vi "GetProperties.vi"(8 "error in":errorcluster, 11 "PageSelector in":refnum<class "PageSelector.lvclass">) -> (0 "error out":errorcluster, 3 "PageSelector out":refnum<class "PageSelector.lvclass">)   [LabVIEW 2014, in "PageSelector.lvclass"]
uses:
  PageSelector.lvclass
  PageSelector.lvclass/PageSelector.ctl
  Control/Control.lvclass
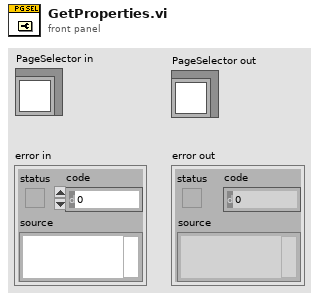
[diagram p1: front panel]
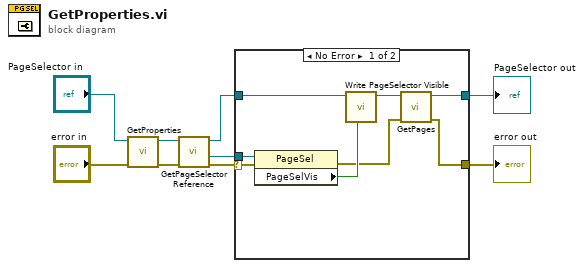
[diagram p0: block diagram]
diagram:
  n1 = call-parent "GetProperties.vi"("error in"="error in", "Control in"="PageSelector in") -> ("error out"=w6:errorcluster, "Control out"=w7:refnum<class "PageSelector.lvclass">)  [unwired: 8 in]
  n2 = call "GetPageSelectorReference.vi"("error in"=w6, "PageSelector in"=w7) -> ("error out"=w5:errorcluster, "page selector reference"=w4:refnum<vi>, "PageSelector out"=w3:refnum<class "PageSelector.lvclass">)  [unwired: 7 in]
  n3 = case shown="No Error" w5 {
    selector: w5 -> [w16 w19]
    tunnel: w4 -> [w15 _]
    tunnel: w3 -> [w17 w18]
    tunnel: [w11 w19] -> w2
    tunnel: [w10 w18] -> w1
    frame No Error {
      n4 = property class="PageSel"(reference=w15, error in=w16) -> (error out=w12:errorcluster, "PageSelVis"=w14:bool)  [unwired: 1 out]
      n5 = call "Write PageSelector Visible.vi"("Visible"=w14, "PageSelector in"=w17) -> ("PageSelector out"=w13:refnum<class "PageSelector.lvclass">)  [unwired: 7 in]
      n6 = call "GetPages.vi"("error in"=w12, "PageSelector in"=w13) -> ("error out"=w11:errorcluster, "PageSelector out"=w10:refnum<class "PageSelector.lvclass">)  [unwired: 8 in]
    }
    frame Error {
    }
  }
  "error out" <- w2
  "PageSelector out" <- w1
